vi "Create.vi"(8 "error in (no error)":errorcluster, 10 "Element":refnum<class "Config Element.lvclass">) -> (0 "error out":errorcluster, 3 "Sequence Constants out":refnum<class "Sequence Constants.lvclass">)   [LabVIEW 2020, in "VolatusSeqConfig.lvlib" / "Sequence Constants.lvclass"]
uses:
  Sequence Constants.lvclass
  Sequence Constants.lvclass/Sequence Constants.ctl
  lv-cdm/CDM-Config/Config Element/Config Element.lvclass
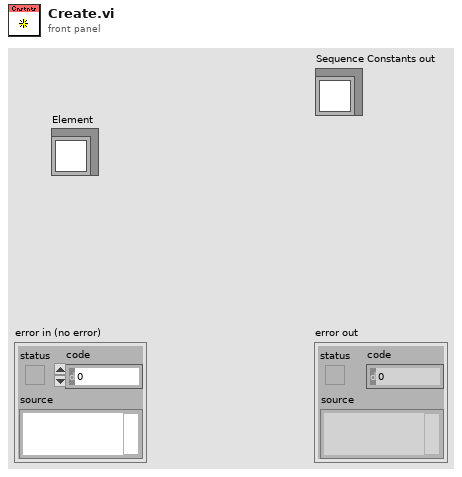
[diagram p1: front panel]
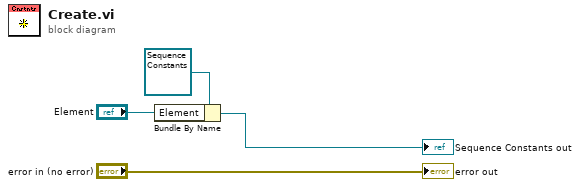
[diagram p0: block diagram]
diagram:
  n1 = Bundle By Name(cluster=refnum<class "Sequence Constants.lvclass"> refnum ("Sequence Constants in"), "Element"="Element") -> (→"Sequence Constants out":refnum<class "Sequence Constants.lvclass">)
  "error out" <- "error in (no error)"
